vi "Enkodery_wolna licz.vi"(7 "Typ (0/1)":i32, 10 "x":dbl[](array[numeric])) -> (2 "Y":dbl)   [LabVIEW 2014]
doc: "wylicza jedną wartość uśrednioną z wektora wejściowego\n0 - mean (wartość środkowa)\n1 - średnia arytmetyczna"
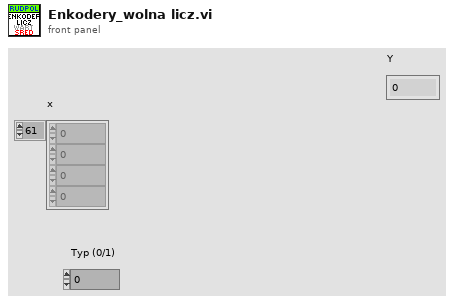
[diagram p1: front panel]
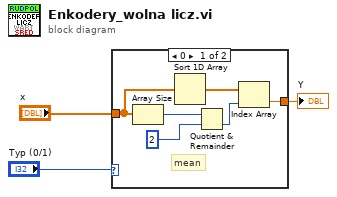
[diagram p0: block diagram]
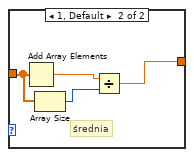
[diagram p2: hidden frame]
diagram:
  n1 = case shown="0" "Typ (0/1)" {
    tunnel: "x" -> [w5 w13]
    tunnel: [w6 w10] -> w1
    frame 0 {
      # "mean"
      n2 = Array Size(array=w5) -> (size(s)=w9:i32)
      n3 = Sort 1D Array(array=w5) -> (sorted array=w4:dbl[])
      n4 = Quotient & Remainder(x=w9, y=2) -> (floor(x/y)=w7:i32)  [unwired: 1 out]
      n5 = Index Array(array=w4, index=w7) -> (element=w6:dbl)
    }
    frame 1, Default {
      # "średnia"
      n6 = Add Array Elements(numeric array=w13) -> (sum=w12:dbl)
      n7 = Array Size(array=w13) -> (size(s)=w11:i32)
      n8 = Divide(x=w12, y=w11) -> (x/y=w10:dbl)
    }
  }
  "Y" <- w1
